vi "Pattern Align(SubVI).vi"(9 "curX(p)":sgl, 10 "defX(p)":sgl, 11 "Range(p)":sgl) -> (0 "In Range?":bool, 1 "Bck":bool, 3 "Fwd":bool)   [LabVIEW 2017]
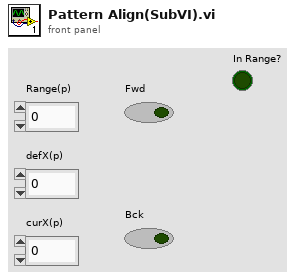
[diagram p1: front panel]
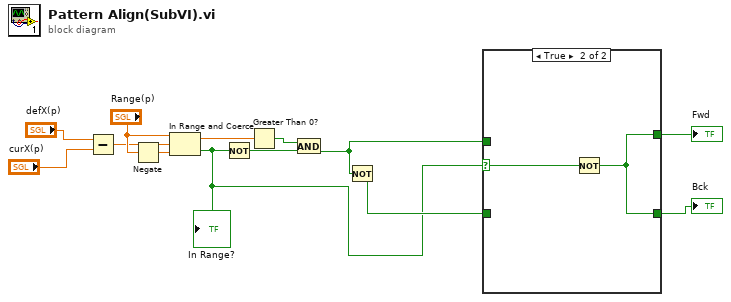
[diagram p0: block diagram]
diagram:
  n1 = Subtract(x="defX(p)", y="curX(p)") -> (x-y=w6:sgl)
  n2 = Negate(x="Range(p)") -> (-x=w8:sgl)
  n3 = In Range and Coerce(upper limit="Range(p)", x=w6, lower limit=w8) -> (coerced(x)=w9:sgl, In Range?=w3:bool)
  "In Range?" <- w3
  n4 = Not(x=w3) -> (.not. x?=w11:bool)
  n5 = Greater Than 0?(x=w9) -> (x > 0?=w10:bool)
  n6 = And(x=w10, y=w11) -> (x .and. y?=w13:bool)
  n7 = Not(x=w13) -> (.not. x?=w12:bool)
  n8 = case shown="True" w3 {
    selector: w3 -> [_ w17]
    tunnel: w13 -> [w15 _]
    tunnel: w12 -> [w14 _]
    tunnel: [w15 w16] -> w2
    tunnel: [w14 w16] -> w1
    frame False {
    }
    frame True {
      n9 = Not(x=w17) -> (.not. x?=w16:bool)
    }
  }
  "Fwd" <- w2
  "Bck" <- w1
